vi "Call ShowErrors Dialog.vi"(8 "error in (no error)":errorcluster, 9 "ErrorList":string[](array[string]), 10 "menubar":refnum<k9>, 11 "Main UI Ref":refnum<vi>) -> (0 "error out":errorcluster)   [LabVIEW 2017, in "ErrorHandler.lvclass"]
doc: "Developed by Kevin Thompson\nkevin@thompsonengineering.net\n\nCopyright 2018\nThompson Engineering, LLC"
uses:
  ErrorHandler.lvclass
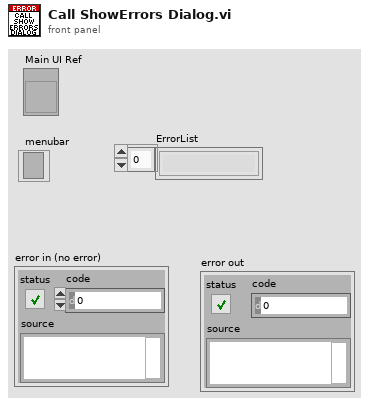
[diagram p1: front panel]
types:
  T1 = enum32{"Bad", "Idle", "Run top level", "Running"}
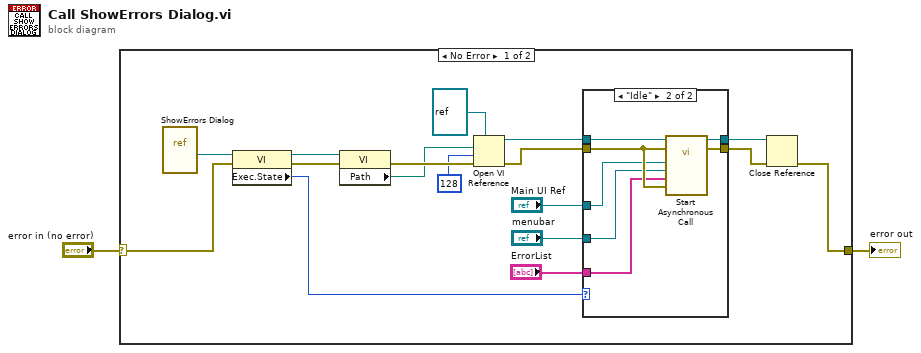
[diagram p0: block diagram]
diagram:
  n1 = case shown="No Error" "error in (no error)" {
    selector: "error in (no error)" -> [w12 w29]
    tunnel: [w18 w29] -> w2
    frame No Error {
      n2 = vi-ref "ShowErrors Dialog.vi"() -> (w9:refnum<vi>)
      n3 = property class="VI"(reference=w9, error in=w12) -> (reference out=w13:refnum<vi>, error out=w16:errorcluster, "Exec.State"=w11:T1)
      n4 = property class="VI"(reference=w13, error in=w16) -> (error out=w17:errorcluster, "Path"=w14:path)  [unwired: 1 out]
      n5 = Open VI Reference(type specifier VI Refnum (for type only)=refnum<vi> refnum, vi path=w14, options=128, error in (no error)=w17) -> (vi reference=w8:refnum<vi>, error out=w10:errorcluster)  [unwired: 2 in]
      n6 = case shown="\"Idle\"" w11 {
        tunnel: [w21 w28] -> w19
        tunnel: w10 -> [w21 w25]
        tunnel: w8 -> [w20 w27]
        tunnel: [w20 w26] -> w7
        tunnel: "menubar" -> [_ w24]
        tunnel: "Main UI Ref" -> [_ w23]
        tunnel: "ErrorList" -> [_ w22]
        frame "Bad", Default {
        }
        frame "Idle" {
          n7 = call-by-ref "Start Asynchronous Call"(reference=w27, error in=w25, 8:"error in (no error)"=w25, "ErrorList"=w22, "menubar"=w24, "Main UI Ref"=w23) -> (reference out=w26:refnum<vi>, error out=w28:errorcluster)  [unwired: 7 in, 1 out]
        }
      }
      n8 = Close Reference(reference=w7, error in (no error)=w19) -> (error out=w18:errorcluster)
    }
    frame Error {
    }
  }
  "error out" <- w2
